vi "Get All SetList Display Info_queue.vi"(0 "SetList Dev queue":refnum<queue>) -> (1 "Invalid Dev queue?":bool, 2 "Columns":refnum<class "Column.lvclass">[](array[class]), 3 "DevNums":i32[](array[numeric]), 4 "Table Data":string[][](array[string]))   [LabVIEW 2013]
uses:
  ColumnVIs/Column/Column.lvclass
  Device/Device.lvclass
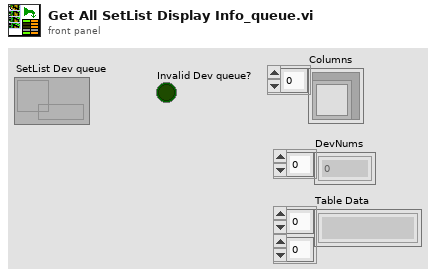
[diagram p1: front panel]
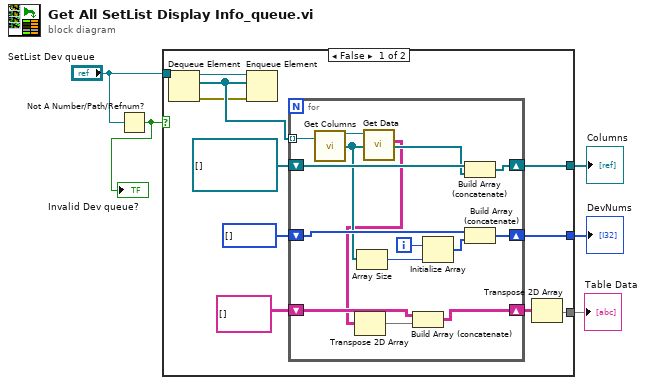
[diagram p0: block diagram]
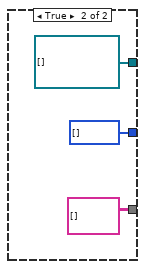
[diagram p2: hidden frame]
diagram:
  n1 = Not A Number/Path/Refnum?(number/path/refnum="SetList Dev queue") -> (NaN/Path/Refnum?=w1:bool)
  "Invalid Dev queue?" <- w1
  n2 = case shown="False" w1 {
    tunnel: [w14 refnum<class "Column.lvclass">[] [] ("Columns")] -> w5
    tunnel: [w13 i32[] []] -> w4
    tunnel: [w10 string[][] []] -> w3
    tunnel: "SetList Dev queue" -> [w9 _]
    frame False {
      n3 = Dequeue Element(queue=w9) -> (queue out=w8:refnum<queue>, element=w7:refnum<class "Device.lvclass">[], error out=w6:errorcluster)  [unwired: 2 in, 1 out]
      n4 = Enqueue Element(queue=w8, element=w7, error in (no error)=w6) -> ()  [unwired: 1 in, 3 out]
      n5 = for {
        tunnel: w7 -> [w30] mode=indexing
        shift-right: [w28] -> w14
        shift-left: refnum<class "Column.lvclass">[] [] ("Columns") -> [w29]
        shift-right: [w23] -> w13
        shift-left: i32[] [] -> [w24]
        shift-right: [w17] -> w11
        shift-left: string[][] [] ("Table Control") -> [w20]
        i -> [w26]
        n6 = call-dynamic "Get Columns.vi"("Device in"=w30) -> ("Device out"=w21:refnum<class "Device.lvclass">, "Columns"=w22:refnum<class "Column.lvclass">[])  [unwired: 1 in, 1 out]
        n7 = Array Size(array=w22) -> (size(s)=w27:i32)
        n8 = call-dynamic "Get Data.vi"("Device in"=w21) -> ("Table Indicator"=w19:string[][])  [unwired: 7 in, 2 out]
        n9 = Transpose 2D Array(2D array=w19) -> (transposed array=w18:string[][])
        n10 = Build Array (concatenate)(w20, w18) -> (w17:string[][])
        n11 = Initialize Array(w26, w27) -> (w25:i32[])
        n12 = Build Array (concatenate)(w29, w22) -> (w28:refnum<class "Column.lvclass">[])
        n13 = Build Array (concatenate)(w24, w25) -> (w23:i32[])
      }
      n14 = Transpose 2D Array(2D array=w11) -> (transposed array=w10:string[][])
    }
    frame True {
    }
  }
  "Columns" <- w5
  "DevNums" <- w4
  "Table Data" <- w3
